vi "Measurement Convertor for Voltage.vi"(2 "Measurement":string, 3 "Expression":string) -> (1 "Value":dbl format="%.2f")   [LabVIEW 2023]
uses:
  <vilib>/regexp/Match Regular Expression.xnode
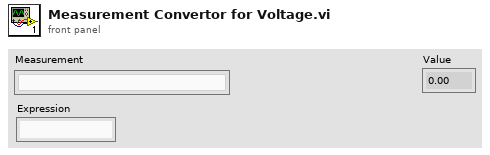
[diagram p1: front panel]
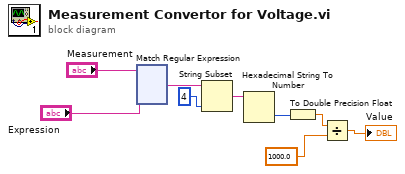
[diagram p0: block diagram]
diagram:
  n1 = xnode "Match Regular Expression"("input string"="Measurement", "regular expression"="Expression") -> ("after match"=w8:string)  [unwired: 4 in, 4 out]
  n2 = String Subset(string=w8, length (rest)=4 ("length (rest)")) -> (substring=w6:string)  [unwired: 1 in]
  n3 = Hexadecimal String To Number(string=w6) -> (number=w3:u32)  [unwired: 2 in, 1 out]
  n4 = To Double Precision Float(number=w3) -> (double precision float=w2:dbl)
  n5 = Divide(x=w2, y=1000.0) -> (x/y=→"Value":dbl)
